vi "configuration UI.vi"() -> ()   [LabVIEW 2013, in "UI Reference editor node.lvclass"]
uses:
  UI Reference editor node.lvclass
  <vilib>/NI/Configuration Framework/Node/NodeRef.ctl
  <vilib>/NI/Configuration Framework/Node/NISE_CEF_Node.lvclass
  <vilib>/NI/AMC/Message Queue.ctl
  <vilib>/NI/AMC/Message.ctl
  <vilib>/NI/Tools/Keyed Array/KeyedArray.ctl
  <vilib>/NI/Configuration Framework/Node/UserEventRef.ctl
  <vilib>/NI/Configuration Framework/Controls/EventCluster.ctl
  module/configuration/UI Reference configuration.lvclass
  <vilib>/NI/Module Execution Interface/Engine Configuration/engine configuration.lvclass
  <vilib>/NI/Tag Bus Data Framework/Configuration Editor/Classes/Engine Parent/Engine Parent Editor Node.lvclass
  <vilib>/NI/Tag Bus/tag/tag descriptor.lvclass
  <vilib>/NI/Tag Bus/tag/Data Type.ctl
  <vilib>/NI/Tag Bus/tag/tag descriptor.lvclass/tag descriptor.ctl
  module/configuration/UI Reference configuration.lvclass/UI Reference configuration.ctl
  UI Reference editor node.lvclass/UI Reference editor node.ctl
  <vilib>/NI/Tag Bus/tag/write tag name.vi
  <vilib>/NI/Tag Bus/tag/write data type.vi
  module/configuration/Read VI name.vi
  <vilib>/NI/Tag Bus Data Framework/Configuration Editor/Classes/Module editor node/Read Module Configuration.vi
  <vilib>/NI/Configuration Framework/serializable configuration/NISE_CEF_serializable configuration.lvclass
  <vilib>/NI/Tag Bus Module Framework/module configuration/TBM module configuration.lvclass
  <vilib>/NI/Configuration Framework/NISE_CEF_TreeControl.lvlib
  <vilib>/NI/Tag Bus Data Framework/Configuration Editor/Classes/Module editor node/module editor node.lvclass
  <vilib>/NI/Tools/Keyed Array/Tools_KeyedArray.lvlib
  <vilib>/NI/AMC/AMC.lvlib
panel:
  in  "Tab Control":enum32{"Static Configuration"}(tab)
  in  "autogen":bool
  in  "browse":bool
  out "UI to Load":string
  in  "hidden_remove":bool
  in  "hidden_settings":bool
  in  "hidden_Add":bool
  in  "Remove Button":bool
  in  "Add Button":bool
  in  "channel":i32(listbox)
  in  "settings":bool
  in  "user event":T1
  in  "main queue":T2
  in  "node ref":T3
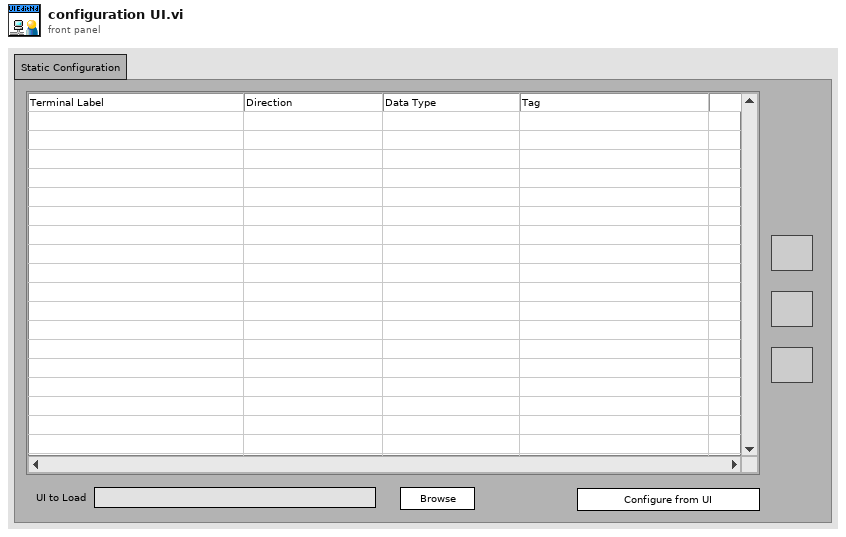
[diagram p1: front panel]
types:
  T1 = typedef "NISE_CEF_Node.lvclass/UserEventRef.ctl" = refnum<user-event>
  T2 = typedef "AMC.lvlib/Message Queue.ctl" = refnum<queue>
  T3 = typedef "NISE_CEF_Node.lvclass/NodeRef.ctl" = refnum<data-value>
  T4 = typedef "NISE_CEF_TreeControl.lvlib/EventCluster.ctl" = cluster{"command":string, "data":string}
  T5 = typedef "tag bus.lvlib/tag descriptor.lvclass/Data Type.ctl" = enum16{"Double", "Single", "I64", "I32", "I16", "I8", "U64", "U32", "U16", "U8", "Boolean", "String", "Array of Double", "Array of Single", "Array of I64", "Array of I32", "Array of I16", "Array of I8", "Array of U64", "Array of U32", "Array of U16", "Array of U8", "Array of Boolean", "Array of String"}
  T6 = typedef "UI Reference editor node.lvclass/table line.ctl" = cluster{"channel":refnum<class "TBM channel.lvclass">, "tag name":string}
  T7 = typedef "LVPoint32TypeDef.ctl" = cluster{"Horizontal":i32, "Vertical":i32}
  T8 = typedef "LVRowAndColumnTypeDef.ctl" = cluster{"Row":i32, "Column":i32}
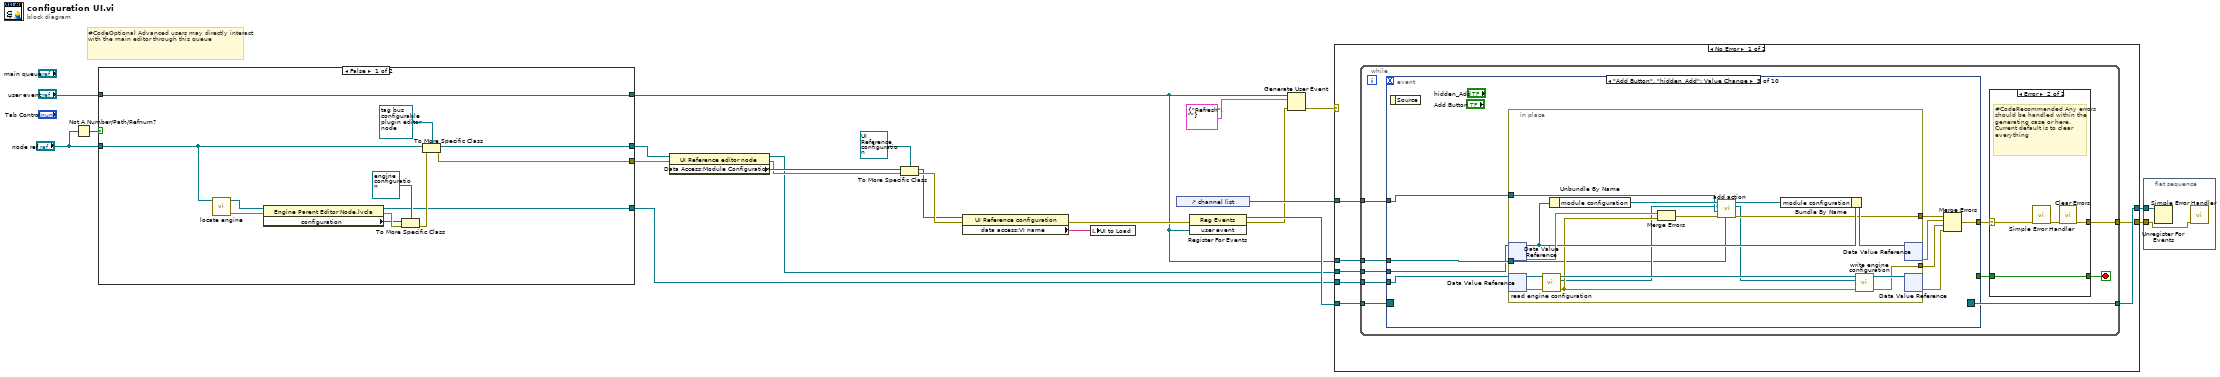
[diagram p0: block diagram]
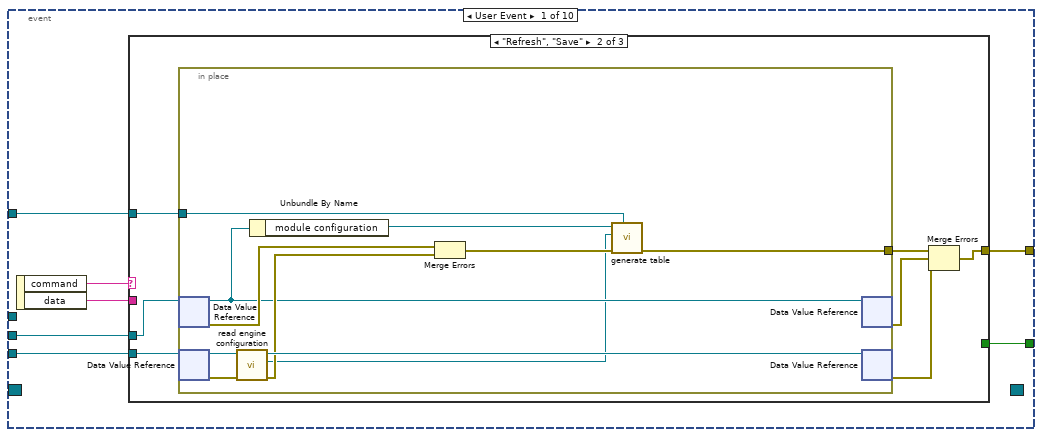
[diagram p3: hidden frame]
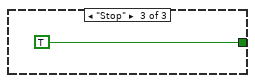
[diagram p5: hidden frame]
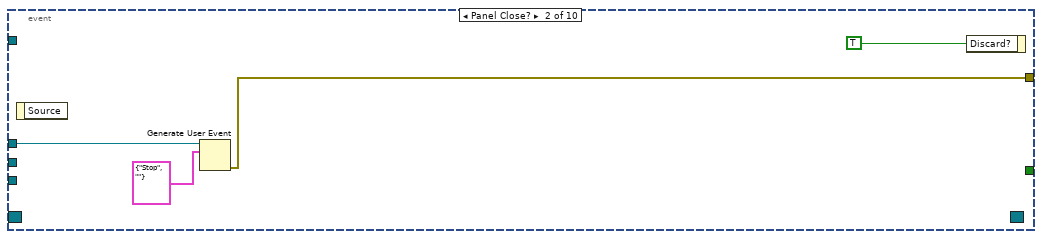
[diagram p6: hidden frame]
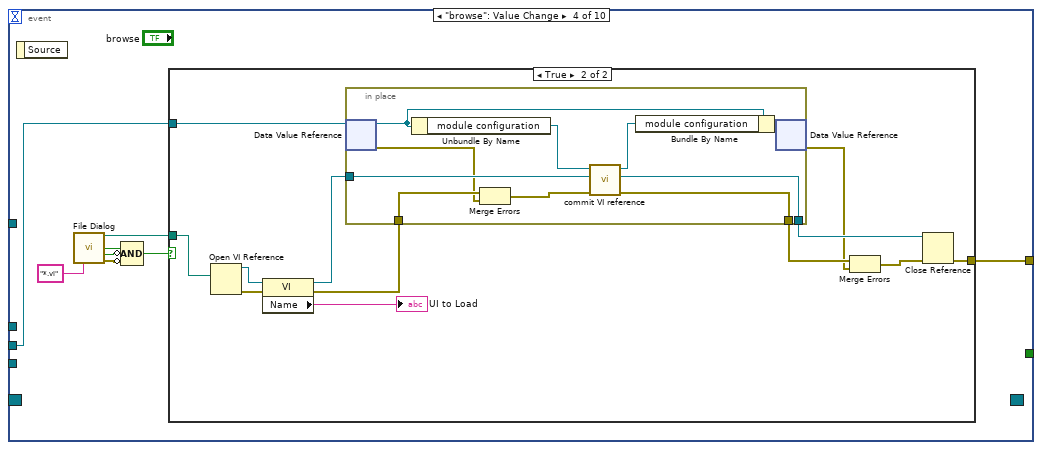
[diagram p7: hidden frame]
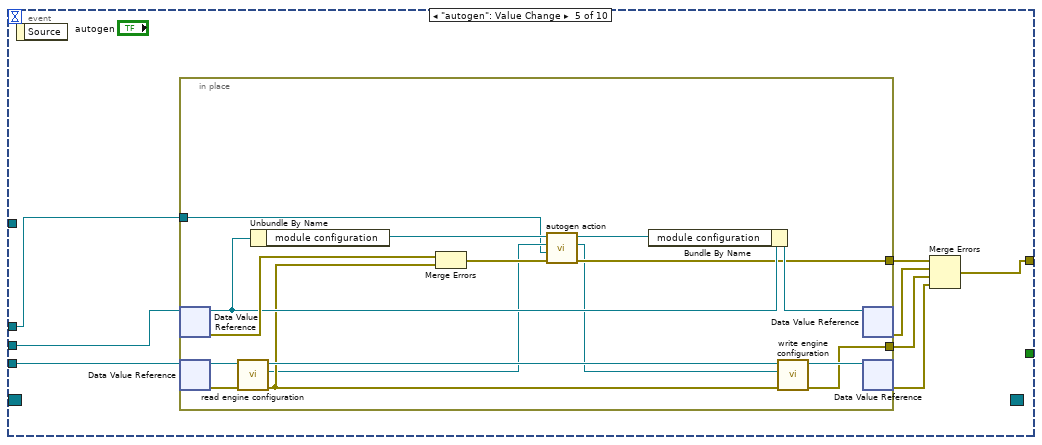
[diagram p9: hidden frame]
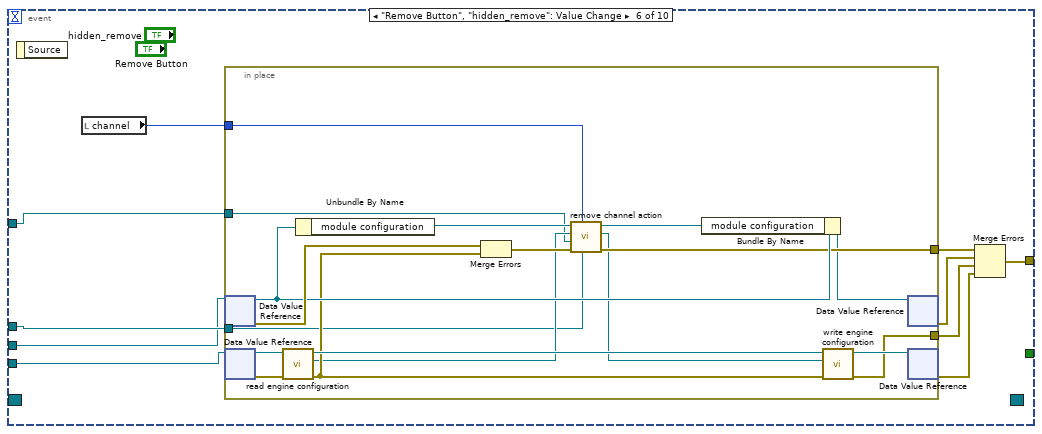
[diagram p10: hidden frame]
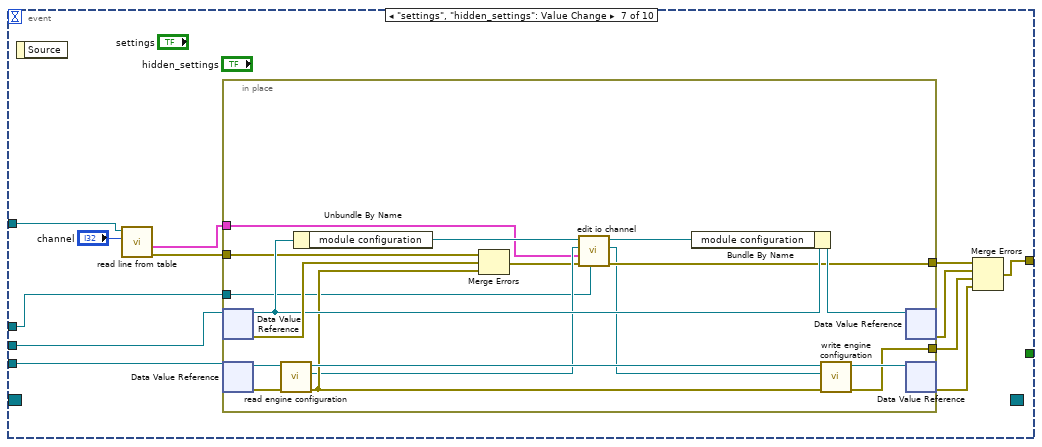
[diagram p11: hidden frame]
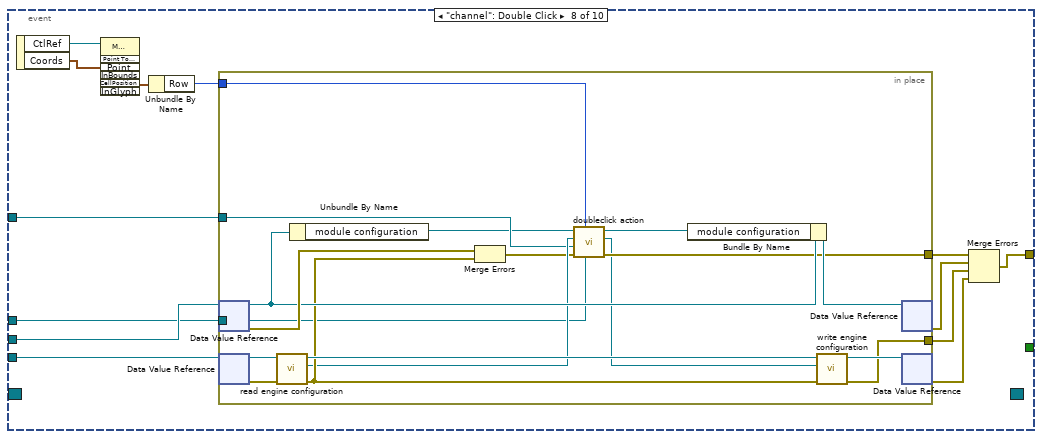
[diagram p12: hidden frame]
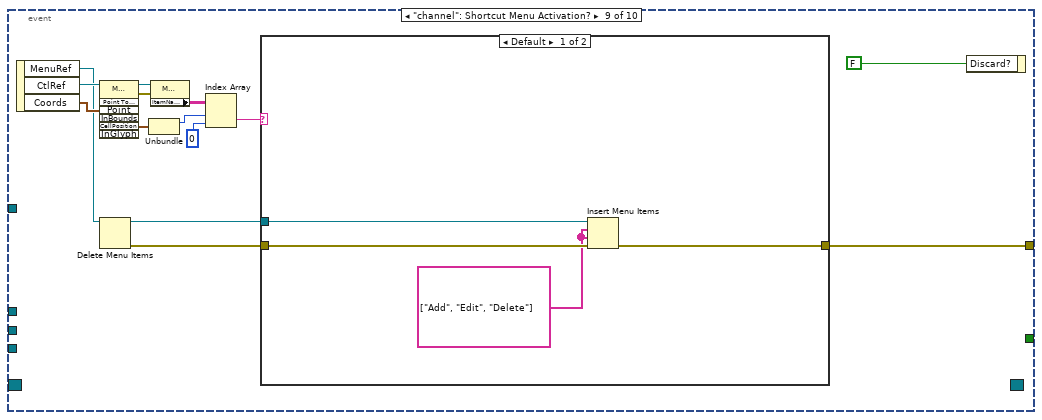
[diagram p13: hidden frame]
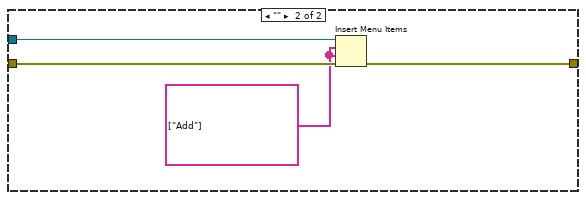
[diagram p14: hidden frame]
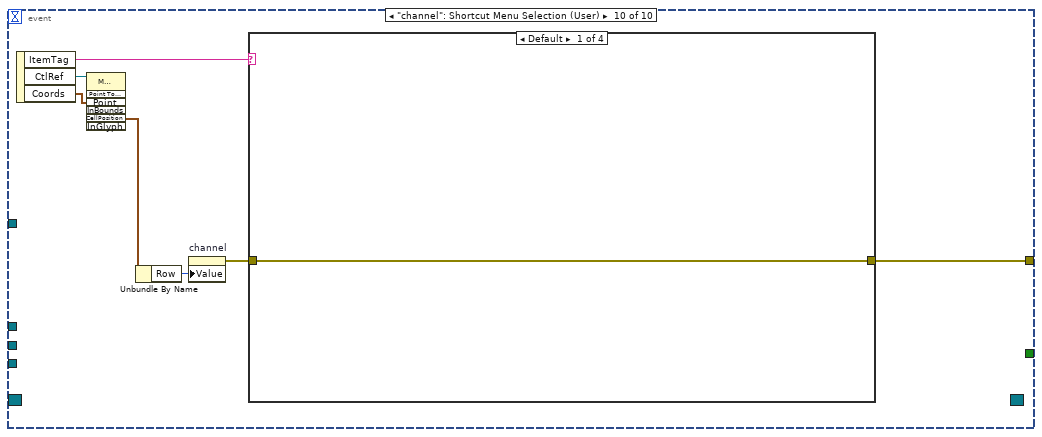
[diagram p15: hidden frame]
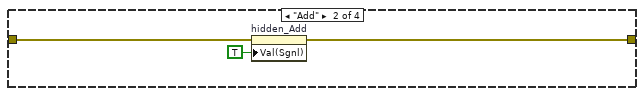
[diagram p16: hidden frame]
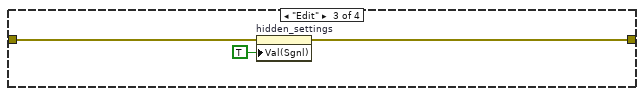
[diagram p17: hidden frame]
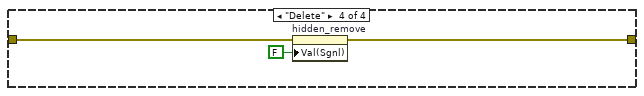
[diagram p18: hidden frame]
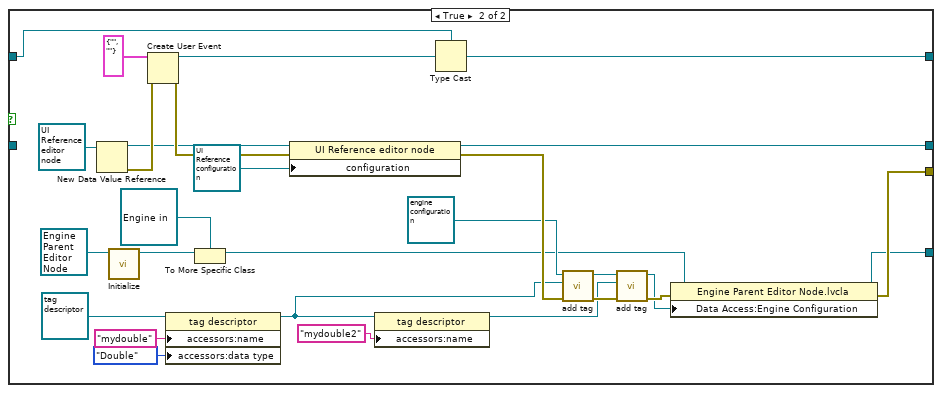
[diagram p20: hidden frame]
diagram:
  # "#CodeOptional Advanced users may directly interact with the main editor through this queue"
  n1 = Not A Number/Path/Refnum?(number/path/refnum="node ref") -> (NaN/Path/Refnum?=w16:bool)
  n2 = case shown="False" w16 {
    tunnel: "user event" -> [w34 w40]
    tunnel: [w34 w41] -> w4
    tunnel: "node ref" -> [w32 _]
    tunnel: [w31 w56] -> w11
    tunnel: [w30 w38] -> w14
    tunnel: [w23 w36] -> w9
    frame False {
      n3 = call <vilib>:"locate engine.vi"("component"=w32) -> ("error out"=w27:errorcluster, "engine"=w29:refnum<data-value>)  [unwired: 9 in]
      n4 = property class="Engine Parent Editor Node.lvcla"(reference=w29, error in=w27) -> (reference out=w23:refnum<data-value>, error out=w26:errorcluster, "configuration"=w25:refnum<class "NISE_CEF_serializable configuration.lvclass">)
      n5 = To More Specific Class(target class=refnum<class "engine configuration.lvclass"> refnum ("engine configuration.lvclass"), reference=w25, error in=w26) -> (error out=w24:errorcluster)  [unwired: 1 out]
      n6 = To More Specific Class(target class=refnum<data-value> refnum ("data value reference"), reference=w32, error in=w24) -> (specific class reference=w31:refnum<data-value>, error out=w30:errorcluster)
    }
    frame True {
      n7 = New Data Value Reference(data value=refnum<class "UI Reference editor node.lvclass"> refnum ("tag bus configurable plugin editor node")) -> (data value reference=w55:refnum<data-value>, error out=w58:errorcluster)  [unwired: 1 in]
      n8 = call-dynamic "Initialize.vi"("Engine in"=refnum<class "Engine Parent Editor Node.lvclass"> refnum) -> ("data value reference"=w54:T3)  [unwired: 8 in, 2 out]
      n9 = Create User Event(user event datatype=T4 {"command"="", "data"=""} ("event data"), error in=w58) -> (user event=w61:refnum<user-event>, error out=w57:errorcluster)
      n10 = property class="tag descriptor"(reference=refnum<class "tag descriptor.lvclass"> refnum ("tag descriptor"), "accessors:name"="mydouble" ("name"), "accessors:data type"=Data_Type."Double" ("data type")) -> (reference out=w42:refnum<class "tag descriptor.lvclass">)  [unwired: 1 in, 1 out]
      n11 = To More Specific Class(target class=refnum<data-value> refnum ("data value reference"), reference=w54) -> (specific class reference=w37:refnum<data-value>)  [unwired: 1 in, 1 out]
      n12 = property class="UI Reference editor node"(reference=w55, error in=w57, "configuration"=refnum<class "UI Reference configuration.lvclass"> refnum ("tag bus configurable plugin module configuration")) -> (reference out=w56:refnum<data-value>, error out=w48:errorcluster)
      n13 = property class="tag descriptor"(reference=w42, "accessors:name"="mydouble2" ("name")) -> (reference out=w43:refnum<class "tag descriptor.lvclass">)  [unwired: 1 in, 1 out]
      n14 = Type Cast(type=w40, x=w61) -> (*(type *) &x=w41:T1)
      n15 = call <vilib>:"add tag.vi"("error in"=w48, "tag descriptor"=w42, "engine configuration in"=refnum<class "engine configuration.lvclass"> refnum ("Engine Configuration")) -> ("error out"=w46:errorcluster, "engine configuration out"=w45:refnum<class "engine configuration.lvclass">)  [unwired: 7 in]
      n16 = call <vilib>:"add tag.vi"("error in"=w46, "tag descriptor"=w43, "engine configuration in"=w45) -> ("error out"=w44:errorcluster, "engine configuration out"=w35:refnum<class "engine configuration.lvclass">)  [unwired: 7 in]
      n17 = property class="Engine Parent Editor Node.lvcla"(reference=w37, error in=w44, "Data Access:Engine Configuration"=w35) -> (reference out=w36:refnum<data-value>, error out=w38:errorcluster)
    }
  }
  n18 = property class="UI Reference editor node"(reference=w11, error in=w14) -> (reference out=w10:refnum<data-value>, error out=w17:errorcluster, "Data Access:Module Configuration"=w18:refnum<class "TBM module configuration.lvclass">)
  n19 = To More Specific Class(target class=refnum<class "UI Reference configuration.lvclass"> refnum ("tag bus configurable plugin module configuration"), reference=w18, error in=w17) -> (specific class reference=w6:refnum<class "UI Reference configuration.lvclass">, error out=w12:errorcluster)
  n20 = property class="UI Reference configuration"(reference=w6, error in=w12) -> (error out=w7:errorcluster, "data access:VI name"=w5:string)  [unwired: 1 out]
  n21 = local write "UI to Load"(w5) -> ()
  n22 = control-ref of="channel list"() -> (w8:refnum<vi>)
  n23 = register-events(error in=w7, w4) -> (reference out=w22:refnum<event-registration>, error out=w2:errorcluster)  [unwired: 1 in]
  n24 = Generate User Event(user event=w4, event data cluster=T4 {"command"="Refresh", "data"=""} ("event data"), error in=w2) -> (error out=w1:errorcluster)  [unwired: 1 in, 1 out]
  n25 = case shown="No Error" w1 {
    selector: w1 -> [_ w324]
    tunnel: w22 -> [w69 w325]
    tunnel: [w68 w325] -> w21
    tunnel: [w67 w324] -> w20
    tunnel: w10 -> [w66 _]
    tunnel: w9 -> [w65 _]
    tunnel: w8 -> [w64 _]
    tunnel: w4 -> [w63 _]
    frame No Error {
      n26 = while {
        tunnel: w69 -> [w79]
        tunnel: [w78] -> w68
        tunnel: w66 -> [w74]
        tunnel: w65 -> [w73]
        tunnel: w63 -> [w72]
        tunnel: w64 -> [w70]
        tunnel: [w75] -> w67
        stop <- w77 stop-if-true
        n27 = event shown="[2] \"Add Button\", \"hidden_Add\": Value Change" {
          selector: w79 -> [_ _ _ _ _ _ _ _ _ _]
          dyn-events: [_ _ _ _ _ _ _ _ _ _] -> w78
          timeout: _ -> [_ _ _ _ _ _ _ _ _ _]
          tunnel: [w92 _ _ _ _ _ _ _ _ _] -> w76
          tunnel: [w87 w112 w120 w143 w175 w201 w229 w259 w285 w310] -> w71
          tunnel: w74 -> [w90 _ w116 w142 w173 w196 w227 w257 _ _]
          tunnel: w73 -> [w89 _ w119 _ w174 w197 w228 w258 _ _]
          tunnel: w72 -> [_ w113 w117 _ w172 w199 w225 w256 _ _]
          tunnel: w70 -> [w86 _ w118 _ _ w198 w234 w255 _ _]
          event User Event {
            n28 = event-data() -> ("command"=w91:string, "data"=w88:string)  [unwired: 1 in]
            n29 = case shown="\"Refresh\", \"Save\"" w91 {
              tunnel: [_ _ TRUE] -> w92
              tunnel: w90 -> [_ w95 _]
              tunnel: w89 -> [_ w96 _]
              tunnel: w88 -> [_ _ _]
              tunnel: [_ w97 _] -> w87
              tunnel: w86 -> [_ w98 _]
              frame Default {
              }
              frame "Refresh", "Save" {
                n30 = in-place {
                  in-place-border: [w110] -> w99
                  in-place-border: w98 -> [w109]
                  n31 = in-place-dvr #1(w95) -> (w102:refnum<class "UI Reference editor node.lvclass">, w103:errorcluster)
                  n32 = in-place-dvr #2(w96) -> (w107:refnum<class "Engine Parent Editor Node.lvclass">, w106:errorcluster)
                  n33 = call <vilib>:"read engine configuration.vi"("error in"=w106, "Engine Parent Editor Node in"=w107) -> ("error out"=w104:errorcluster, "engine configuration"=w100:refnum<class "engine configuration.lvclass">, "Engine Parent Editor Node out"=w105:refnum<class "Engine Parent Editor Node.lvclass">)  [unwired: 7 in]
                  n34 = Unbundle By Name(w102) -> ("module configuration"=w101:refnum<class "UI Reference configuration.lvclass">)
                  n35 = Merge Errors(w103, w104) -> (w108:errorcluster)
                  n36 = call "generate table.vi"("table"=w109, "error in"=w108, "engine configuration"=w100, "tag bus configurable plugin module configuration"=w101) -> ("error out"=w110:errorcluster)  [unwired: 7 in]
                  n37 = in-place-dvr #1(w102) -> (w93:errorcluster)  [unwired: 1 out]
                  n38 = in-place-dvr #2(w105) -> (w94:errorcluster)  [unwired: 1 out]
                }
                n39 = Merge Errors(w99, w93, w94) -> (w97:errorcluster)
              }
              frame "Stop" {
              }
            }
          }
          event Panel Close? {
            n40 = event-data() -> ()  [unwired: 1 in, 1 out]
            n41 = Generate User Event(user event=w113, event data cluster=T4 {"command"="Stop", "data"=""} ("event data")) -> (error out=w112:errorcluster)  [unwired: 2 in, 1 out]
            n42 = event-data("Discard?"=TRUE) -> ()  [unwired: 1 in, 1 out]
          }
          event "Add Button", "hidden_Add": Value Change {
            n43 = event-data() -> ()  [unwired: 1 in, 1 out]
            n44 = in-place {
              in-place-border: [w132] -> w121
              in-place-border: [w135] -> w124
              in-place-border: w118 -> [w127]
              in-place-border: w117 -> [w125]
              n45 = in-place-dvr #3(w116) -> (w138:refnum<class "UI Reference editor node.lvclass">, w139:errorcluster)
              n46 = in-place-dvr #4(w119) -> (w141:refnum<class "Engine Parent Editor Node.lvclass">, w140:errorcluster)
              n47 = call <vilib>:"read engine configuration.vi"("error in"=w140, "Engine Parent Editor Node in"=w141) -> ("error out"=w134:errorcluster, "engine configuration"=w126:refnum<class "engine configuration.lvclass">, "Engine Parent Editor Node out"=w137:refnum<class "Engine Parent Editor Node.lvclass">)  [unwired: 7 in]
              n48 = Unbundle By Name(w138) -> ("module configuration"=w128:refnum<class "UI Reference configuration.lvclass">)
              n49 = Merge Errors(w139, w134) -> (w131:errorcluster)
              n50 = call "add action.vi"("user event"=w125, "error in"=w131, "channel list"=w127, "engine configuration in"=w126, "UI Reference configuration in"=w128) -> ("error out"=w132:errorcluster, "engine configuration out"=w129:refnum<class "engine configuration.lvclass">, "UI Reference configuration out"=w130:refnum<class "UI Reference configuration.lvclass">)  [unwired: 4 in]
              n51 = Bundle By Name(cluster=w138, "module configuration"=w130) -> (w133:refnum<class "UI Reference editor node.lvclass">)
              n52 = call <vilib>:"write engine configuration.vi"("error in"=w134, "engine configuration"=w129, "Engine Parent Editor Node in"=w137) -> ("error out"=w135:errorcluster, "Engine Parent Editor Node out"=w136:refnum<class "Engine Parent Editor Node.lvclass">)  [unwired: 7 in]
              n53 = in-place-dvr #3(w133) -> (w123:errorcluster)  [unwired: 1 out]
              n54 = in-place-dvr #4(w136) -> (w122:errorcluster)  [unwired: 1 out]
            }
            n55 = Merge Errors(w121, w123, w124, w122) -> (w120:errorcluster)
          }
          event "browse": Value Change {
            n56 = event-data() -> ()  [unwired: 1 in, 1 out]
            n57 = call "File Dialog"("pattern (all files)"="*.vi") -> ("selected path"=w144:path, "exists"=w148:bool, "cancelled"=w147:bool, "error out"=w146:errorcluster)  [unwired: 11 in]
            n58 = Compound Arithmetic op=AND(w148, invert w147, invert w146) -> (w145:bool)
            n59 = case shown="True" w145 {
              tunnel: w144 -> [_ w161]
              tunnel: [_ w157] -> w143
              tunnel: w142 -> [_ w152]
              frame False {
              }
              frame True {
                n60 = Open VI Reference(vi path=w161) -> (vi reference=w159:refnum<vi>, error out=w160:errorcluster)  [unwired: 5 in]
                n61 = property class="VI"(reference=w159, error in=w160) -> (reference out=w154:refnum<vi>, error out=w155:errorcluster, "Name"=→"UI to Load":string)
                n62 = in-place {
                  in-place-border: [w171] -> w156
                  in-place-border: w155 -> [w170]
                  in-place-border: w154 -> [w169]
                  in-place-border: [w168] -> w153
                  n63 = in-place-dvr #5(w152) -> (w165:refnum<class "UI Reference editor node.lvclass">, w162:errorcluster)
                  n64 = Unbundle By Name(w165) -> ("module configuration"=w167:refnum<class "UI Reference configuration.lvclass">)
                  n65 = Merge Errors(w170, w162) -> (w163:errorcluster)
                  n66 = call "commit VI reference.vi"("error in"=w163, "VI Refnum in"=w169, "UI Reference configuration in"=w167) -> ("error out"=w168:errorcluster, "VI Refnum out"=w171:refnum<vi>, "UI Reference configuration out"=w164:refnum<class "UI Reference configuration.lvclass">)  [unwired: 6 in]
                  n67 = Bundle By Name(cluster=w165, "module configuration"=w164) -> (w166:refnum<class "UI Reference editor node.lvclass">)
                  n68 = in-place-dvr #5(w166) -> (w150:errorcluster)  [unwired: 1 out]
                }
                n69 = Merge Errors(w153, w150) -> (w151:errorcluster)
                n70 = Close Reference(reference=w156, error in (no error)=w151) -> (error out=w157:errorcluster)
              }
            }
          }
          event "autogen": Value Change {
            n71 = event-data() -> ()  [unwired: 1 in, 1 out]
            n72 = in-place {
              in-place-border: [w186] -> w176
              in-place-border: [w189] -> w179
              in-place-border: w172 -> [w180]
              n73 = in-place-dvr #6(w173) -> (w192:refnum<class "UI Reference editor node.lvclass">, w193:errorcluster)
              n74 = in-place-dvr #7(w174) -> (w195:refnum<class "Engine Parent Editor Node.lvclass">, w194:errorcluster)
              n75 = call <vilib>:"read engine configuration.vi"("error in"=w194, "Engine Parent Editor Node in"=w195) -> ("error out"=w188:errorcluster, "engine configuration"=w184:refnum<class "engine configuration.lvclass">, "Engine Parent Editor Node out"=w191:refnum<class "Engine Parent Editor Node.lvclass">)  [unwired: 7 in]
              n76 = Unbundle By Name(w192) -> ("module configuration"=w183:refnum<class "UI Reference configuration.lvclass">)
              n77 = Merge Errors(w193, w188) -> (w185:errorcluster)
              n78 = call "autogen action.vi"("error in"=w185, "user event"=w180, "engine configuration in"=w184, "UI Reference configuration in"=w183) -> ("error out"=w186:errorcluster, "engine configuration out"=w181:refnum<class "engine configuration.lvclass">, "UI Reference configuration out"=w182:refnum<class "UI Reference configuration.lvclass">)  [unwired: 5 in]
              n79 = Bundle By Name(cluster=w192, "module configuration"=w182) -> (w187:refnum<class "UI Reference editor node.lvclass">)
              n80 = call <vilib>:"write engine configuration.vi"("error in"=w188, "engine configuration"=w181, "Engine Parent Editor Node in"=w191) -> ("error out"=w189:errorcluster, "Engine Parent Editor Node out"=w190:refnum<class "Engine Parent Editor Node.lvclass">)  [unwired: 7 in]
              n81 = in-place-dvr #6(w187) -> (w178:errorcluster)  [unwired: 1 out]
              n82 = in-place-dvr #7(w190) -> (w177:errorcluster)  [unwired: 1 out]
            }
            n83 = Merge Errors(w176, w178, w179, w177) -> (w175:errorcluster)
          }
          event "Remove Button", "hidden_remove": Value Change {
            n84 = event-data() -> ()  [unwired: 1 in, 1 out]
            n85 = local read "channel"() -> (w200:i32)
            n86 = in-place {
              in-place-border: [w215] -> w202
              in-place-border: [w217] -> w205
              in-place-border: w200 -> [w210]
              in-place-border: w199 -> [w209]
              in-place-border: w198 -> [w208]
              n87 = in-place-dvr #8(w196) -> (w220:refnum<class "UI Reference editor node.lvclass">, w221:errorcluster)
              n88 = in-place-dvr #9(w197) -> (w223:refnum<class "Engine Parent Editor Node.lvclass">, w222:errorcluster)
              n89 = call <vilib>:"read engine configuration.vi"("error in"=w222, "Engine Parent Editor Node in"=w223) -> ("error out"=w216:errorcluster, "engine configuration"=w213:refnum<class "engine configuration.lvclass">, "Engine Parent Editor Node out"=w219:refnum<class "Engine Parent Editor Node.lvclass">)  [unwired: 7 in]
              n90 = Unbundle By Name(w220) -> ("module configuration"=w211:refnum<class "UI Reference configuration.lvclass">)
              n91 = Merge Errors(w221, w216) -> (w214:errorcluster)
              n92 = call "remove channel action.vi"("user event"=w209, "channel"=w210, "error in"=w214, "channel list"=w208, "engine configuration in"=w213, "UI Reference configuration in"=w211) -> ("error out"=w215:errorcluster, "engine configuration out"=w212:refnum<class "engine configuration.lvclass">, "UI Reference configuration out"=w206:refnum<class "UI Reference configuration.lvclass">)  [unwired: 3 in]
              n93 = Bundle By Name(cluster=w220, "module configuration"=w206) -> (w207:refnum<class "UI Reference editor node.lvclass">)
              n94 = call <vilib>:"write engine configuration.vi"("error in"=w216, "engine configuration"=w212, "Engine Parent Editor Node in"=w219) -> ("error out"=w217:errorcluster, "Engine Parent Editor Node out"=w218:refnum<class "Engine Parent Editor Node.lvclass">)  [unwired: 7 in]
              n95 = in-place-dvr #8(w207) -> (w204:errorcluster)  [unwired: 1 out]
              n96 = in-place-dvr #9(w218) -> (w203:errorcluster)  [unwired: 1 out]
            }
            n97 = Merge Errors(w202, w204, w205, w203) -> (w201:errorcluster)
          }
          event "settings", "hidden_settings": Value Change {
            n98 = event-data() -> ()  [unwired: 1 in, 1 out]
            n99 = call "read line from table.vi"("line number"="channel", "channels table"=w234) -> ("error out"=w226:errorcluster, "line"=w224:T6)  [unwired: 6 in, 2 out]
            n100 = in-place {
              in-place-border: [w243] -> w230
              in-place-border: [w247] -> w233
              in-place-border: w226 -> [w244]
              in-place-border: w225 -> [w237]
              in-place-border: w224 -> [w236]
              n101 = in-place-dvr #10(w227) -> (w250:refnum<class "UI Reference editor node.lvclass">, w251:errorcluster)
              n102 = in-place-dvr #11(w228) -> (w253:refnum<class "Engine Parent Editor Node.lvclass">, w252:errorcluster)
              n103 = call <vilib>:"read engine configuration.vi"("error in"=w252, "Engine Parent Editor Node in"=w253) -> ("error out"=w246:errorcluster, "engine configuration"=w239:refnum<class "engine configuration.lvclass">, "Engine Parent Editor Node out"=w249:refnum<class "Engine Parent Editor Node.lvclass">)  [unwired: 7 in]
              n104 = Unbundle By Name(w250) -> ("module configuration"=w240:refnum<class "UI Reference configuration.lvclass">)
              n105 = Merge Errors(w244, w251, w246) -> (w238:errorcluster)
              n106 = call "edit io channel.vi"("user event"=w237, "error in"=w238, "line"=w236, "engine configuration in"=w239, "tag bus configurable plugin module configuration in"=w240) -> ("error out"=w243:errorcluster, "engine configuration"=w241:refnum<class "engine configuration.lvclass">, "tag bus configurable plugin module configuration out"=w242:refnum<class "UI Reference configuration.lvclass">)  [unwired: 4 in]
              n107 = Bundle By Name(cluster=w250, "module configuration"=w242) -> (w245:refnum<class "UI Reference editor node.lvclass">)
              n108 = call <vilib>:"write engine configuration.vi"("error in"=w246, "engine configuration"=w241, "Engine Parent Editor Node in"=w249) -> ("error out"=w247:errorcluster, "Engine Parent Editor Node out"=w248:refnum<class "Engine Parent Editor Node.lvclass">)  [unwired: 7 in]
              n109 = in-place-dvr #10(w245) -> (w232:errorcluster)  [unwired: 1 out]
              n110 = in-place-dvr #11(w248) -> (w231:errorcluster)  [unwired: 1 out]
            }
            n111 = Merge Errors(w230, w232, w233, w231) -> (w229:errorcluster)
          }
          event "channel": Double Click {
            n112 = event-data() -> ("CtlRef"=w266:refnum<vi>, "Coords"=w265:T7)  [unwired: 1 in]
            n113 = invoke class="MCListbox (strict)" method="Point To Row Column"(reference=w266, "Point"=w265) -> ("CellPosition"=w264:T8)  [unwired: 5 in, 6 out]
            n114 = Unbundle By Name(w264) -> ("Row"=w254:i32)
            n115 = in-place {
              in-place-border: [w275] -> w260
              in-place-border: [w278] -> w263
              in-place-border: w256 -> [w271]
              in-place-border: w255 -> [w270]
              in-place-border: w254 -> [w268]
              n116 = in-place-dvr #12(w257) -> (w281:refnum<class "UI Reference editor node.lvclass">, w282:errorcluster)
              n117 = in-place-dvr #13(w258) -> (w284:refnum<class "Engine Parent Editor Node.lvclass">, w283:errorcluster)
              n118 = call <vilib>:"read engine configuration.vi"("error in"=w283, "Engine Parent Editor Node in"=w284) -> ("error out"=w277:errorcluster, "engine configuration"=w272:refnum<class "engine configuration.lvclass">, "Engine Parent Editor Node out"=w280:refnum<class "Engine Parent Editor Node.lvclass">)  [unwired: 7 in]
              n119 = Unbundle By Name(w281) -> ("module configuration"=w269:refnum<class "UI Reference configuration.lvclass">)
              n120 = Merge Errors(w282, w277) -> (w267:errorcluster)
              n121 = call "doubleclick action.vi"("user event"=w271, "Row"=w268, "error in"=w267, "channel list"=w270, "engine configuration in"=w272, "UI Reference configuration in"=w269) -> ("error out"=w275:errorcluster, "engine configuration out"=w273:refnum<class "engine configuration.lvclass">, "UI Reference configuration out"=w274:refnum<class "UI Reference configuration.lvclass">)  [unwired: 3 in]
              n122 = Bundle By Name(cluster=w281, "module configuration"=w274) -> (w276:refnum<class "UI Reference editor node.lvclass">)
              n123 = call <vilib>:"write engine configuration.vi"("error in"=w277, "engine configuration"=w273, "Engine Parent Editor Node in"=w280) -> ("error out"=w278:errorcluster, "Engine Parent Editor Node out"=w279:refnum<class "Engine Parent Editor Node.lvclass">)  [unwired: 7 in]
              n124 = in-place-dvr #12(w276) -> (w262:errorcluster)  [unwired: 1 out]
              n125 = in-place-dvr #13(w279) -> (w261:errorcluster)  [unwired: 1 out]
            }
            n126 = Merge Errors(w260, w262, w263, w261) -> (w259:errorcluster)
          }
          event "channel": Shortcut Menu Activation? {
            n127 = event-data() -> ("MenuRef"=w295:refnum<k9>, "CtlRef"=w297:refnum<vi>, "Coords"=w296:T7)  [unwired: 1 in]
            n128 = invoke class="MCListbox (strict)" method="Point To Row Column"(reference=w297, "Point"=w296) -> (reference out=w294:refnum<vi>, error out=w293:errorcluster, "CellPosition"=w292:T8)  [unwired: 5 in, 4 out]
            n129 = Delete Menu Items(9:w295) -> (0:w286:errorcluster, 3:w287:refnum<k9>)  [unwired: 3 in]
            n130 = Unbundle(w292) -> ("Row"=w290:i32)  [unwired: 1 out]
            n131 = property class="MCListbox (strict)"(reference=w294, error in=w293) -> ("ItemNames"=w291:string[][])  [unwired: 2 out]
            n132 = Index Array(array=w291, index (row)=w290, index (col)=0 ("disabled index (col)")) -> (element=w288:string)
            n133 = case shown="Default" w288 {
              tunnel: w287 -> [w302 w306]
              tunnel: w286 -> [w301 w305]
              tunnel: [w300 w304] -> w285
              frame Default {
                w299 = string[] ["Add", "Edit", "Delete"] ("item names")
                n134 = Insert Menu Items(6:w301, 7:w299, 8:w299, 9:w302) -> (0:w300:errorcluster)  [unwired: 2 in, 2 out]
              }
              frame "" {
                w303 = string[] ["Add"] ("item names")
                n135 = Insert Menu Items(6:w305, 7:w303, 8:w303, 9:w306) -> (0:w304:errorcluster)  [unwired: 2 in, 2 out]
              }
            }
            n136 = event-data("Discard?"=FALSE) -> ()  [unwired: 1 in, 1 out]
          }
          event "channel": Shortcut Menu Selection (User) {
            n137 = event-data() -> ("ItemTag"=w311:string, "CtlRef"=w312:refnum<vi>, "Coords"=w313:T7)  [unwired: 1 in]
            n138 = invoke class="MCListbox (strict)" method="Point To Row Column"(reference=w312, "Point"=w313) -> ("CellPosition"=w308:T8)  [unwired: 5 in, 6 out]
            n139 = Unbundle By Name(w308) -> ("Row"=w307:i32)
            n140 = property on="channel" class="MCListbox (strict)"("Value"=w307) -> (error out=w309:errorcluster)  [unwired: 2 in, 1 out]
            n141 = case shown="Default" w311 {
              tunnel: w309 -> [w314 w316 w320 w323]
              tunnel: [w314 w315 w319 w322] -> w310
              frame Default {
              }
              frame "Add" {
                n142 = property on="hidden_Add" class="Bool (strict)"(error in=w316, "Val(Sgnl)"=TRUE ("Value (Signaling)")) -> (error out=w315:errorcluster)  [unwired: 1 in, 1 out]
              }
              frame "Edit" {
                n143 = property on="hidden_settings" class="Bool (strict)"(error in=w320, "Val(Sgnl)"=TRUE ("Value (Signaling)")) -> (error out=w319:errorcluster)  [unwired: 1 in, 1 out]
              }
              frame "Delete" {
                n144 = property on="hidden_remove" class="Bool (strict)"(error in=w323, "Val(Sgnl)"=FALSE ("Value (Signaling)")) -> (error out=w322:errorcluster)  [unwired: 1 in, 1 out]
              }
            }
          }
        }
        n145 = case shown="Error" w71 {
          selector: w71 -> [w80 w84]
          tunnel: [w81 w85] -> w77
          tunnel: w76 -> [w81 w85]
          tunnel: [w80 w82] -> w75
          frame No Error {
          }
          frame Error {
            # "#CodeRecommended Any errors should be handled within the generating case or here. Current default is to clear everything"
            n146 = call <vilib>:"Simple Error Handler.vi"("error in (no error)"=w84) -> ("error out"=w83:errorcluster)  [unwired: 4 in, 4 out]
            n147 = call <vilib>:"Clear Errors.vi"("error in (no error)"=w83) -> ("error out"=w82:errorcluster)  [unwired: 6 in]
          }
        }
      }
    }
    frame Error {
    }
  }
  n148 = flat-sequence {
    tunnel: w21 -> [w327]
    tunnel: w20 -> [w326]
    frame #0 {
      n149 = Unregister For Events(event registration refnum=w327) -> ()  [unwired: 1 in, 1 out]
      n150 = call <vilib>:"Simple Error Handler.vi"("error in (no error)"=w326) -> ()  [unwired: 4 in, 5 out]
    }
  }
